vi "Read System Configurations.vi"   [LabVIEW 2014, in "Associated Power Technologies 8500 Series.lvlib"]
uses:
  <instrlib>/Associated Power Technologies 8500 Series/Associated Power Technologies 8500 Series.lvlib
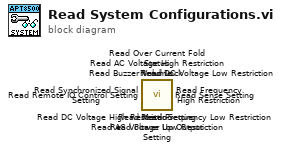
[diagram p0: block diagram]
diagram:
  n1 = call <instrlib>:"Read Meter Setting.vi"() -> ()  [unwired: 9 in, 3 out]
  n2 = call <instrlib>:"Read Lock.vi"() -> ()  [unwired: 9 in, 3 out]
  n3 = call <instrlib>:"Read Synchronized Signal Setting.vi"() -> ()  [unwired: 9 in, 3 out]
  n4 = call <instrlib>:"Read Sense Setting.vi"() -> ()  [unwired: 9 in, 3 out]
  n5 = call <instrlib>:"Read Power Up Output Setting.vi"() -> ()  [unwired: 9 in, 3 out]
  n6 = call <instrlib>:"Read Over Current Fold Status.vi"() -> ()  [unwired: 9 in, 3 out]
  n7 = call <instrlib>:"Read Buzzer Volume.vi"() -> ()  [unwired: 9 in, 3 out]
  n8 = call <instrlib>:"Read Frequency Low Restriction.vi"() -> ()  [unwired: 9 in, 3 out]
  n9 = call <instrlib>:"Read Frequency High Restriction.vi"() -> ()  [unwired: 9 in, 3 out]
  n10 = call <instrlib>:"Read DC Voltage Low Restriction.vi"() -> ()  [unwired: 9 in, 3 out]
  n11 = call <instrlib>:"Read DC Voltage High Restriction.vi"() -> ()  [unwired: 9 in, 3 out]
  n12 = call <instrlib>:"Read AC Voltage Low Restriction.vi"() -> ()  [unwired: 9 in, 3 out]
  n13 = call <instrlib>:"Read AC Voltage High Restriction.vi"() -> ()  [unwired: 9 in, 3 out]
  n14 = call <instrlib>:"Read Remote IO Control Setting.vi"() -> ()  [unwired: 9 in, 3 out]
